vi "Compare Multiple Channel Values.vi"(6 "Values":dbl[](array[numeric]), 7 "Expected Values":dbl[](array[numeric]), 8 "error in (no error)":errorcluster, 9 "Scalar Outputs":string[](array[string]), 10 "Scalar Inputs":string[](array[string]), 11 ".NET Refnum in":T1) -> (0 "error out":errorcluster, 2 "Equals?":bool)   [LabVIEW 2026, in "FPGA Addon Speciality IO Tests.lvclass"]
uses:
  FPGA Addon Speciality IO Tests.lvclass
  <vilib>/NI VeriStand/Execution/Workspace/NI_VS Workspace ExecutionAPI.lvlib
  <vilib>/NI VeriStand/Execution/Workspace/NI VeriStand - Set Multiple Channel Values.vi
  <vilib>/NI VeriStand/Execution/Workspace/NI VeriStand - Get Multiple Channel Values.vi
  <vilib>/NI VeriStand/Execution/Workspace/WorkspaceAPI.ctl
  C:/Users/Administrator/Desktop/Jatin/All DNC DLLs/NationalInstruments.VeriStand.ClientAPI.dll
  Jatin/All DNC DLLs/NationalInstruments.VeriStand.ClientAPI.dll
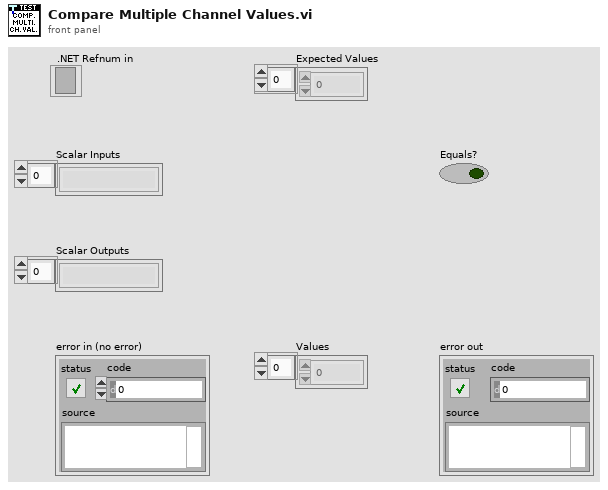
[diagram p1: front panel]
types:
  T1 = typedef "NI_VS Workspace ExecutionAPI.lvlib/WorkspaceAPI.ctl" = refnum<k39>
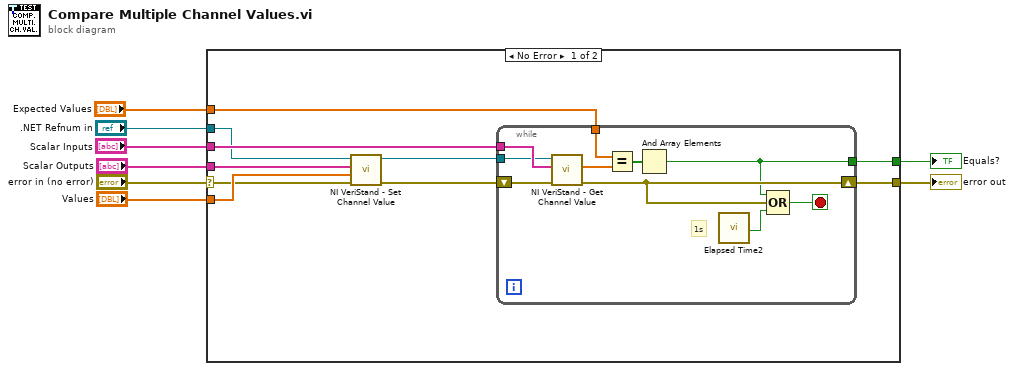
[diagram p0: block diagram]
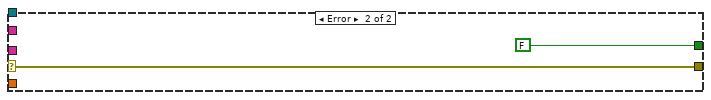
[diagram p2: hidden frame]
diagram:
  n1 = case shown="No Error" "error in (no error)" {
    selector: "error in (no error)" -> [w10 w29]
    tunnel: "Expected Values" -> [w18 _]
    tunnel: [w17 w29] -> w7
    tunnel: [w9 FALSE] -> w6
    tunnel: "Scalar Inputs" -> [w15 _]
    tunnel: "Values" -> [w13 _]
    tunnel: "Scalar Outputs" -> [w12 _]
    tunnel: ".NET Refnum in" -> [w11 _]
    frame No Error {
      n2 = call-poly <vilib>:"NI VeriStand - Set Channel Value.vi"("error in (no error)"=w10, "Values"=w13, "Channels"=w12, "WorkspaceManager in"=w11) -> ("error out"=w16:errorcluster, "WorkspaceManager out"=w14:T1)  [unwired: 6 in]
      n3 = while {
        tunnel: w18 -> [w28]
        tunnel: w15 -> [w25]
        tunnel: w14 -> [w24]
        shift-right: [w21] -> w17
        shift-left: w16 -> [w26]
        tunnel: [w19] -> w9
        stop <- w20 stop-if-true
        # "1s"
        n4 = call-poly <vilib>:"NI VeriStand - Get Channel Value.vi"("error in (no error)"=w26, "Channels"=w25, "WorkspaceManager in"=w24) -> ("error out"=w21:errorcluster, "Values"=w27:dbl[])  [unwired: 6 in, 1 out]
        n5 = Equal?(x=w28, y=w27) -> (x = y?=w22:bool[])
        n6 = And Array Elements(Boolean array=w22) -> (logical AND=w19:bool)
        n7 = call "Elapsed Time2"() -> ("Time has Elapsed"=w23:bool)  [unwired: 12 in, 7 out]
        n8 = Compound Arithmetic op=OR(w19, w21, w23) -> (w20:bool)
      }
    }
    frame Error {
    }
  }
  "error out" <- w7
  "Equals?" <- w6
